vi "Analyse.vi"(8 "error in (no error)":errorcluster, 10 "ImageData":T1, 11 "TemperatureAnalyser in":refnum<class "TemperatureAnalyser.lvclass">) -> (0 "error out":errorcluster, 3 "TemperatureAnalyser out":refnum<class "TemperatureAnalyser.lvclass">)   [LabVIEW 2009, in "Tools.lvlib" / "Imaging.lvlib" / "TemperatureAnalyser.lvclass"]
uses:
  TemperatureAnalyser.lvclass
  TemperatureAnalyser.lvclass/TemperatureAnalyser.ctl
  ImageAnalyser.lvclass
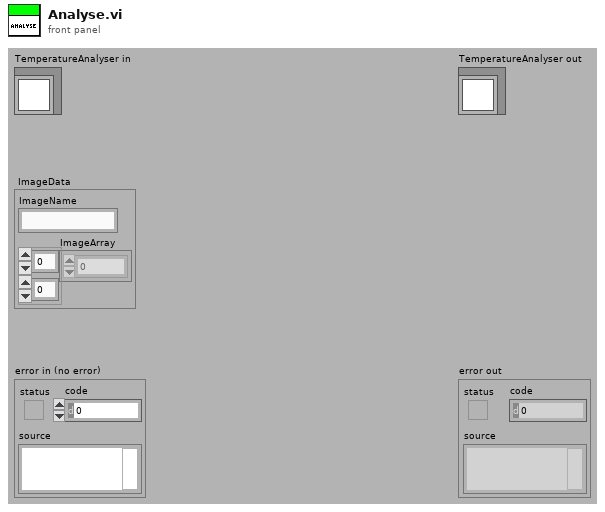
[diagram p1: front panel]
types:
  T1 = cluster{"ImageName":string, "ImageArray":sgl[][]}
  T2 = enum16{"Absorption", "Fluorescence", "Light Sheet", "Dark Ground"}
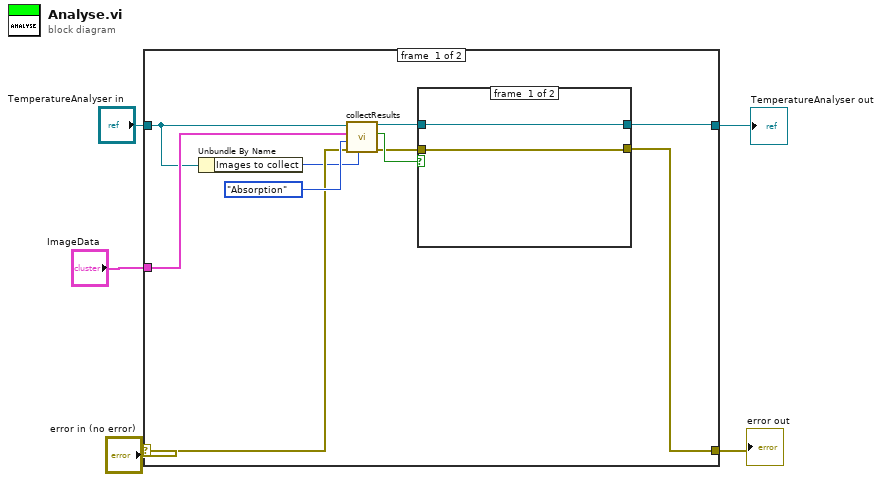
[diagram p0: block diagram]
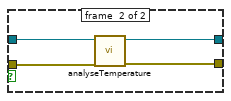
[diagram p2: hidden frame]
diagram:
  n1 = case shown="No Error" "error in (no error)" {
    selector: "error in (no error)" -> [w12 w22]
    tunnel: "TemperatureAnalyser in" -> [w14 w23]
    tunnel: [w7 w23] -> w3
    tunnel: [w6 w22] -> w2
    tunnel: "ImageData" -> [w15 _]
    frame #0 {
      n2 = Unbundle By Name(w14) -> ("Images to collect"=w11:i32)
      n3 = call "collectResults.vi"("Images to Collect"=w11, "error in (no error)"=w12, "Enum"=T2."Absorption", "ImageData"=w15, "ImageAnalyser in"=w14) -> ("error out"=w8:errorcluster, "finished?"=w10:bool, "ImageAnalyser out"=w9:refnum<class "TemperatureAnalyser.lvclass">)  [unwired: 4 in]
      n4 = case shown="True" w10 {
        tunnel: w9 -> [w17 w21]
        tunnel: w8 -> [w16 w20]
        tunnel: [w17 w19] -> w7
        tunnel: [w16 w18] -> w6
        frame #0 {
        }
        frame #1 {
          n5 = call "analyseTemperature.vi"("error in (no error)"=w20, "TemperatureAnalyser in"=w21) -> ("error out"=w18:errorcluster, "TemperatureAnalyser out"=w19:refnum<class "TemperatureAnalyser.lvclass">)  [unwired: 8 in]
        }
      }
    }
    frame #1 {
    }
  }
  "error out" <- w2
  "TemperatureAnalyser out" <- w3
